vi "Rx.vi"(8 "error in (no error)":errorcluster, 10 "Command Parameters":T1, 11 "Dispatcher in":refnum<class "Dispatcher Thread.lvclass">) -> (0 "error out":errorcluster, 3 "Dispatcher out":refnum<class "Dispatcher Thread.lvclass">)   [LabVIEW 2019, in "DSF Core.lvlib" / "Dispatcher Thread.lvclass"]
uses:
  Dispatcher Thread.lvclass
  Interface/Dispatcher/Parameters.ctl
  Dispatcher Thread.lvclass/Dispatcher Thread.ctl
  Interface/Plugin/Command.ctl
  Interface/Dispatcher/Rx Parameters.ctl
  Interface/Interface.lvclass/Interface.ctl
  Interface/Plugin/Send.vi
  Interface/Plugin/Send Plugin Command.vi
  Interface/Send Command.vi
  Interface/Errors.vi
  Interface/Dispatcher/Command Timeout.vi
  Interface/Plugin/Class Name.vi
  Interface/Write RT FIFO.vi
  Interface/New Interface Error.vi
  <vilib>/NI/Memory Manager/VIs/New Error Cluster.vi
  <vilib>/NI/Memory Manager/VIs/New Error Cluster (512B).vi
  <vilib>/NI/Memory Manager/VIs/Set Error Code.vi
  <vilib>/NI/Memory Manager/VIs/Set Error Status.vi
  <vilib>/NI/Memory Manager/VIs/Set Error Source.vi
  <vilib>/NI/Memory Manager/VIs/Write String to Source.vi
  Interface/Interface Error Info.vi
  VIs/Constants/Constants.vi
  VIs/Constants/Base Error Code.vi
  Interface/Interface Error Offset.vi
  Interface/Plugin/Plugin Interface.lvclass
  C:/Dev/GitHub/niveristand-data-sharing-framework-custom-device/Core/Classes/Interface/Interface.lvclass
  VIs/VI Name.vi
  Interface/Dispatcher/Dispatcher Interface.lvclass
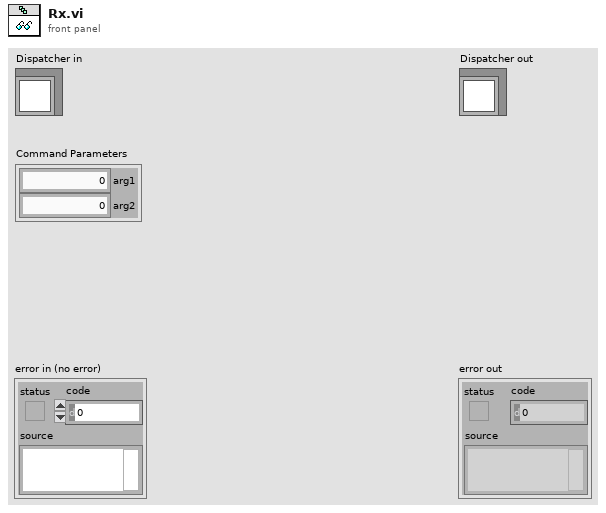
[diagram p1: front panel]
types:
  T1 = typedef "DSF Core.lvlib/Dispatcher Interface.lvclass/Parameters.ctl" = cluster{"arg1":u64, "arg2":u64}
  T2 = typedef "DSF Core.lvlib/Plugin Interface.lvclass/Command.ctl" = enum8{"Idle", "Start", "Set Inline Buffer", "Rx", "Tx", "Shutdown", "Error"}
  T3 = typedef "DSF Core.lvlib/Dispatcher Interface.lvclass/Rx Parameters.ctl" = cluster{"Plugin ID":u8, "Transfer Group ID":u8, "unused long":u16, "Late Count":i32, "Iteration":u64}
  T4 = typedef "DSF Core.lvlib/Dispatcher Thread.lvclass/Plugin Settings.ctl" = cluster{"Transfer Group threads":i32[], "Plugin Thread Interfaces":refnum<class "Plugin Interface.lvclass">[]}
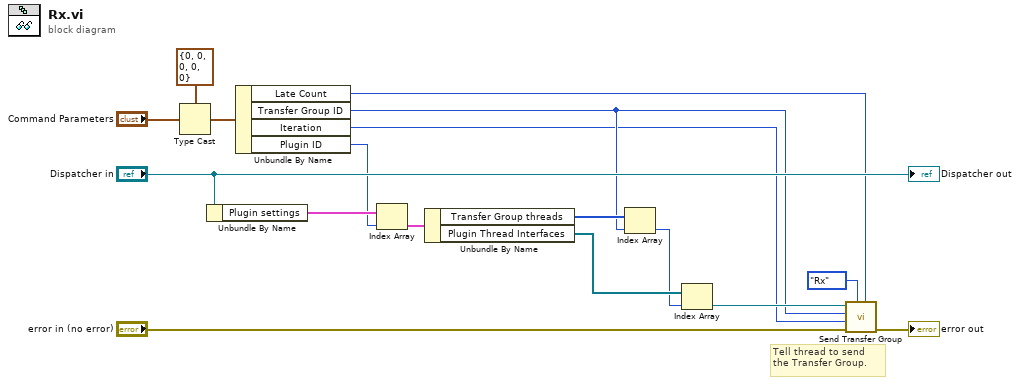
[diagram p0: block diagram]
diagram:
  # "Tell thread to send the Transfer Group."
  n1 = Type Cast(type=T3 {"Plugin ID"=0, "Transfer Group ID"=0, "unused long"=0, "Late Count"=0, "Iteration"=0}, x="Command Parameters") -> (*(type *) &x=w15:T3)
  n2 = Unbundle By Name("Dispatcher in") -> ("Plugin settings"=w14:T4[])
  n3 = Unbundle By Name(w15) -> ("Late Count"=w2:i32, "Transfer Group ID"=w7:u8, "Iteration"=w6:u64, "Plugin ID"=w13:u8)
  n4 = Index Array(array=w14, index=w13) -> (element=w12:T4)
  n5 = Unbundle By Name(w12) -> ("Transfer Group threads"=w11:i32[], "Plugin Thread Interfaces"=w10:refnum<class "Plugin Interface.lvclass">[])
  n6 = Index Array(array=w11, index=w7) -> (element=w1:i32)
  n7 = Index Array(array=w10, index=w1) -> (element=w9:refnum<class "Plugin Interface.lvclass">)
  n8 = call "Send Transfer Group.vi"("Late Count"=w2, "Command"=Command."Rx", "error in (no error)"="error in (no error)", "Transfer Group iteration"=w6, "Transfer Group ID"=w7, "Plugin Interface in"=w9) -> ("error out"=→"error out":errorcluster)  [unwired: 4 in, 1 out]
  "Dispatcher out" <- "Dispatcher in"
